vi "Initialize Hardware References.vi"(8 "error in (no error)":errorcluster, 11 "Hardware Resources in":T1) -> (0 "error out":errorcluster, 3 "Hardware Resources out":T1)   [LabVIEW 2013, in "Acquisition.lvlib"]
doc: "Initialize the hardware references."
uses:
  Acquisition.lvlib
  Hardware Configuration.ctl
  C:/Program Files (x86)/National Instruments/LabVIEW 2013/vi.lib/ULx/ULx_LV.dll
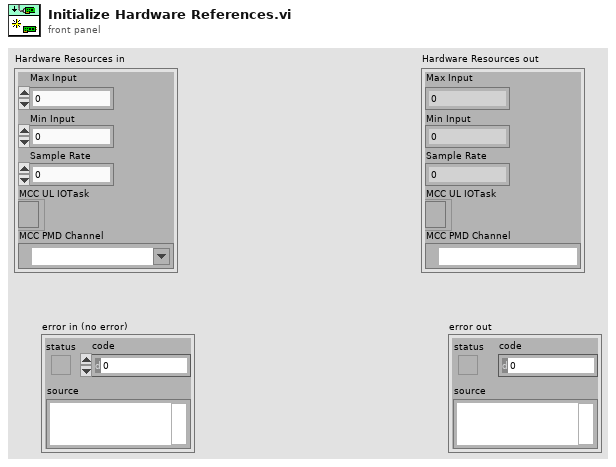
[diagram p1: front panel]
types:
  T1 = typedef "Acquisition.lvlib/Hardware Configuration.ctl" = cluster{"Max Input":dbl, "Min Input":dbl, "Sample Rate":dbl, "MCC UL IOTask":refnum<k24>, "MCC PMD Channel":refnum<k21>}
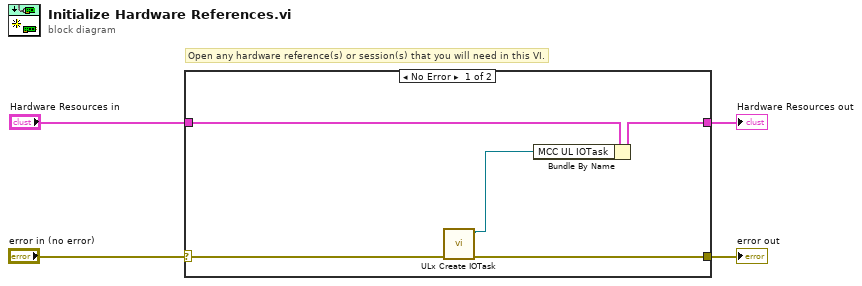
[diagram p0: block diagram]
diagram:
  # "Open any hardware reference(s) or session(s) that you will need in this VI."
  n1 = case shown="No Error" "error in (no error)" {
    selector: "error in (no error)" -> [w5 w10]
    tunnel: [w6 w10] -> w3
    tunnel: "Hardware Resources in" -> [w8 w11]
    tunnel: [w9 w11] -> w1
    frame No Error {
      n2 = call <vilib>:"ULx Create IOTask.vi"("error in"=w5) -> ("error out"=w6:errorcluster, "i/o task out"=w7:refnum<k24>)  [unwired: 9 in]
      n3 = Bundle By Name(cluster=w8, "MCC UL IOTask"=w7) -> (w9:T1)
    }
    frame Error {
    }
  }
  "Hardware Resources out" <- w1
  "error out" <- w3
